vi "MecaOdometry_Reset.vi"(8 "POSE":T3={"TRANSLATION"={"X"=0.0, "Y"=0.0}, "ROTATION"={"VALUE"=0.0, "COS"=1.0, "SIN"=0.0}} {"ROTATION"."SIN" format="%13.4f"; "ROTATION"."COS" format="%13.4f"; "ROTATION"."VALUE" format="%13.4f"; "TRANSLATION"."Y" format="%14.3f"; "TRANSLATION"."X" format="%14.3f"}, 9 "WheelPositions":T1 {"RearRight" format="%19.3f"; "RearLeft" format="%19.3f"; "FrontRight" format="%19.3f"; "FrontLeft" format="%19.3f"}, 10 "GyroOffset":T5 {"SIN" format="%13.4f"; "COS" format="%13.4f"; "VALUE" format="%13.4f"}, 11 "in MECA_DRIVE_ODOMETRY":T2={"POSE"={"TRANSLATION"={"X"=0.0, "Y"=0.0}, "ROTATION"={"VALUE"=0.0, "COS"=1.0, "SIN"=0.0}}, "GyroOffset"={"VALUE"=0.0, "COS"=0.0, "SIN"=0.0}, "PreviousAngle"={"VALUE"=0.0, "COS"=0.0, "SIN"=0.0}, "Kinematics"={"FrontLeft"={"X"=0.0, "Y"=0.0}, "FrontRight"={"X"=0.0, "Y"=0.0}, "RearLeft"={"X"=0.0, "Y"=0.0}, "RearRight"={"X"=0.0, "Y"=0.0}, "InverseKinematics"=[[0.0, 1.0, -1.0, 0.0], [0.0, 1.0, 1.0, 0.0], [0.0, 1.0, 1.0, 0.0], [0.0, 1.0, -1.0, 0.0]], "ForwardKinematics"=[[0.0, 1.0, -1.0, 0.0], [0.0, 1.0, 1.0, 0.0], [0.0, 1.0, 1.0, 0.0], [0.0, 1.0, -1.0, 0.0]], "PrevCoR"={"X"=0.0, "Y"=0.0}}, "PreviousWheelPositions"={"FrontLeft"=0.0, "FrontRight"=0.0, "RearLeft"=0.0, "RearRight"=0.0, "P"=FALSE}} {"PreviousWheelPositions"."RearRight" format="%19.3f"; "PreviousWheelPositions"."RearLeft" format="%19.3f"; "PreviousWheelPositions"."FrontRight" format="%19.3f"; "PreviousWheelPositions"."FrontLeft" format="%19.3f"; "Kinematics"."PrevCoR"."Y" format="%14.3f"; "Kinematics"."PrevCoR"."X" format="%14.3f"; "Kinematics"."RearRight"."Y" format="%14.3f"; "Kinematics"."RearRight"."X" format="%14.3f"; "Kinematics"."RearLeft"."Y" format="%14.3f"; "Kinematics"."RearLeft"."X" format="%14.3f"; "Kinematics"."FrontRight"."Y" format="%14.3f"; "Kinematics"."FrontRight"."X" format="%14.3f"; "Kinematics"."FrontLeft"."Y" format="%14.3f"; "Kinematics"."FrontLeft"."X" format="%14.3f"; "PreviousAngle"."SIN" format="%13.4f"; "PreviousAngle"."COS" format="%13.4f"; "PreviousAngle"."VALUE" format="%13.4f"; "GyroOffset"."SIN" format="%13.4f"; "GyroOffset"."COS" format="%13.4f"; "GyroOffset"."VALUE" format="%13.4f"; "POSE"."ROTATION"."SIN" format="%13.4f"; "POSE"."ROTATION"."COS" format="%13.4f"; "POSE"."ROTATION"."VALUE" format="%13.4f"; "POSE"."TRANSLATION"."Y" format="%14.3f"; "POSE"."TRANSLATION"."X" format="%14.3f"}) -> (3 "out MECA_DRIVE_ODOMETRY":T2={"POSE"={"TRANSLATION"={"X"=0.0, "Y"=0.0}, "ROTATION"={"VALUE"=0.0, "COS"=1.0, "SIN"=0.0}}, "GyroOffset"={"VALUE"=0.0, "COS"=0.0, "SIN"=0.0}, "PreviousAngle"={"VALUE"=0.0, "COS"=0.0, "SIN"=0.0}, "Kinematics"={"FrontLeft"={"X"=0.0, "Y"=0.0}, "FrontRight"={"X"=0.0, "Y"=0.0}, "RearLeft"={"X"=0.0, "Y"=0.0}, "RearRight"={"X"=0.0, "Y"=0.0}, "InverseKinematics"=[[0.0, 1.0, -1.0, 0.0], [0.0, 1.0, 1.0, 0.0], [0.0, 1.0, 1.0, 0.0], [0.0, 1.0, -1.0, 0.0]], "ForwardKinematics"=[[0.0, 1.0, -1.0, 0.0], [0.0, 1.0, 1.0, 0.0], [0.0, 1.0, 1.0, 0.0], [0.0, 1.0, -1.0, 0.0]], "PrevCoR"={"X"=0.0, "Y"=0.0}}, "PreviousWheelPositions"={"FrontLeft"=0.0, "FrontRight"=0.0, "RearLeft"=0.0, "RearRight"=0.0, "P"=FALSE}} {"PreviousWheelPositions"."RearRight" format="%19.3f"; "PreviousWheelPositions"."RearLeft" format="%19.3f"; "PreviousWheelPositions"."FrontRight" format="%19.3f"; "PreviousWheelPositions"."FrontLeft" format="%19.3f"; "Kinematics"."PrevCoR"."Y" format="%14.3f"; "Kinematics"."PrevCoR"."X" format="%14.3f"; "Kinematics"."RearRight"."Y" format="%14.3f"; "Kinematics"."RearRight"."X" format="%14.3f"; "Kinematics"."RearLeft"."Y" format="%14.3f"; "Kinematics"."RearLeft"."X" format="%14.3f"; "Kinematics"."FrontRight"."Y" format="%14.3f"; "Kinematics"."FrontRight"."X" format="%14.3f"; "Kinematics"."FrontLeft"."Y" format="%14.3f"; "Kinematics"."FrontLeft"."X" format="%14.3f"; "PreviousAngle"."SIN" format="%13.4f"; "PreviousAngle"."COS" format="%13.4f"; "PreviousAngle"."VALUE" format="%13.4f"; "GyroOffset"."SIN" format="%13.4f"; "GyroOffset"."COS" format="%13.4f"; "GyroOffset"."VALUE" format="%13.4f"; "POSE"."ROTATION"."SIN" format="%13.4f"; "POSE"."ROTATION"."COS" format="%13.4f"; "POSE"."ROTATION"."VALUE" format="%13.4f"; "POSE"."TRANSLATION"."Y" format="%14.3f"; "POSE"."TRANSLATION"."X" format="%14.3f"})   [LabVIEW 2019, in "Trajectory_Library.lvlib"]
doc: "Resets the robot's position on the field.\n\nThe gyroscope angle does not need to be reset here on the user's robot code. The library automatically takes care of offsetting the gyro angle.\n \nParameters\n - MecaDriveOdometry - Data structure\n - gyroOffset - The angle reported by the gyroscope.\n - wheelPositions -- The distances driven by each wheel.\n - pose - The position on the field that your robot is at. (Meters)\n \nReturns:\n - MecaDriveOdometry - Updated ata structure"
uses:
  Trajectory_Library.lvlib
  TypeDef/TRANSLATION2D.ctl
  TypeDef/ROTATION2D.ctl
  TypeDef/POSE2D.ctl
  TypeDef/MECA_DRIVE_ODOMETRY.ctl
  <vilib>/Analysis/Matrix/Datatypes/RealMatrix.ctl
  <vilib>/Analysis/Matrix/NI_Matrix.lvlib
  TypeDef/MECA_DRIVE_KINEMATICS.ctl
  TypeDef/MECA_WHEEL_POSITIONS.ctl
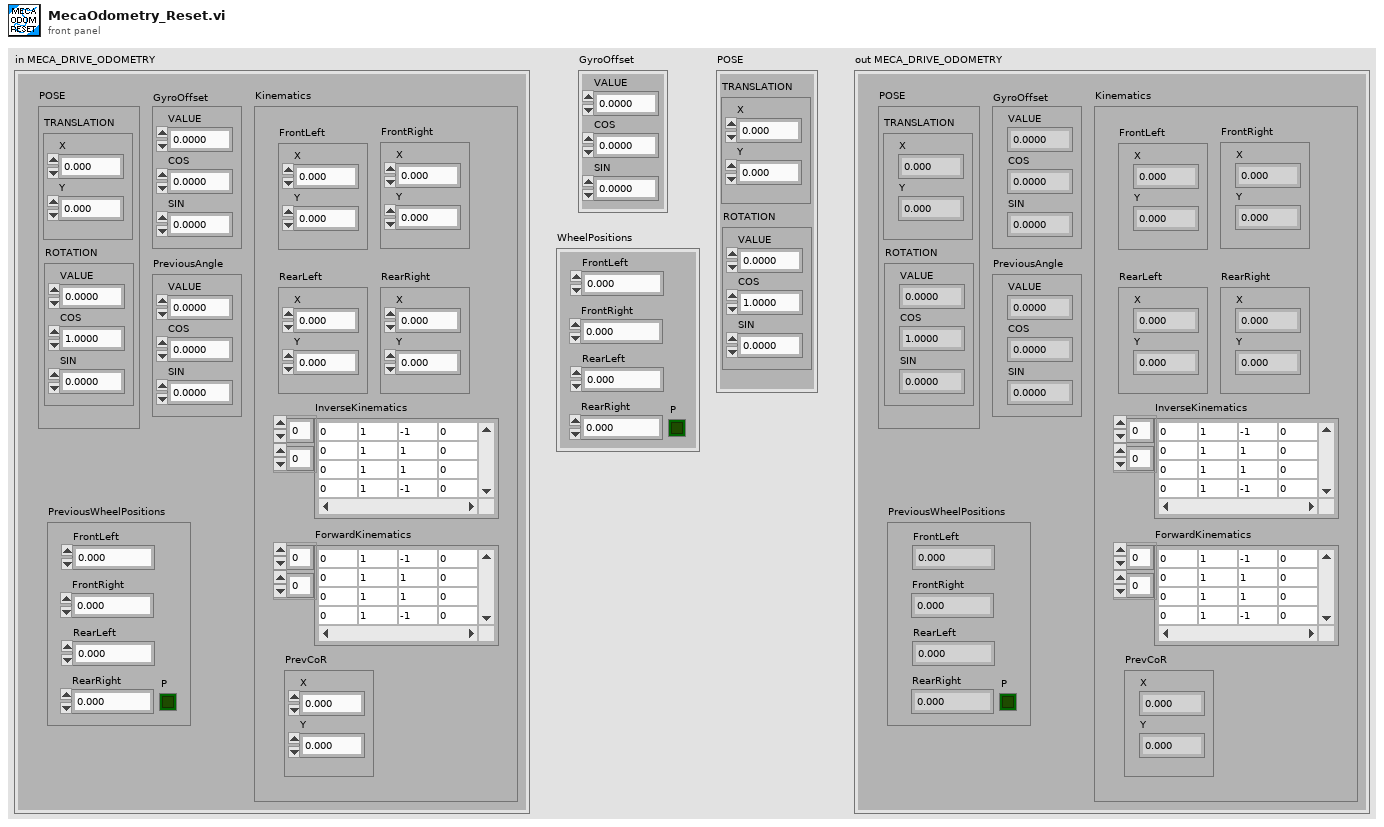
[diagram p1: front panel]
types:
  T1 = typedef "Trajectory_Library.lvlib/MECA_WHEEL_POSITIONS.ctl" = cluster{"FrontLeft":dbl, "FrontRight":dbl, "RearLeft":dbl, "RearRight":dbl, "P":bool}
  T2 = typedef "Trajectory_Library.lvlib/MECA_DRIVE_ODOMETRY.ctl" = cluster{"POSE":T3, "GyroOffset":T5, "PreviousAngle":T5, "Kinematics":T6, "PreviousWheelPositions":T1}
  T3 = typedef "Trajectory_Library.lvlib/POSE2D.ctl" = cluster{"TRANSLATION":T4, "ROTATION":T5}
  T4 = typedef "Trajectory_Library.lvlib/TRANSLATION2D.ctl" = cluster{"X":dbl, "Y":dbl}
  T5 = typedef "Trajectory_Library.lvlib/ROTATION2D.ctl" = cluster{"VALUE":dbl, "COS":dbl, "SIN":dbl}
  T6 = typedef "Trajectory_Library.lvlib/MECA_DRIVE_KINEMATICS.ctl" = cluster{"FrontLeft":T4, "FrontRight":T4, "RearLeft":T4, "RearRight":T4, "InverseKinematics":T7, "ForwardKinematics":T7, "PrevCoR":T4}
  T7 = typedef "NI_Matrix.lvlib/RealMatrix.ctl" = dbl[][]
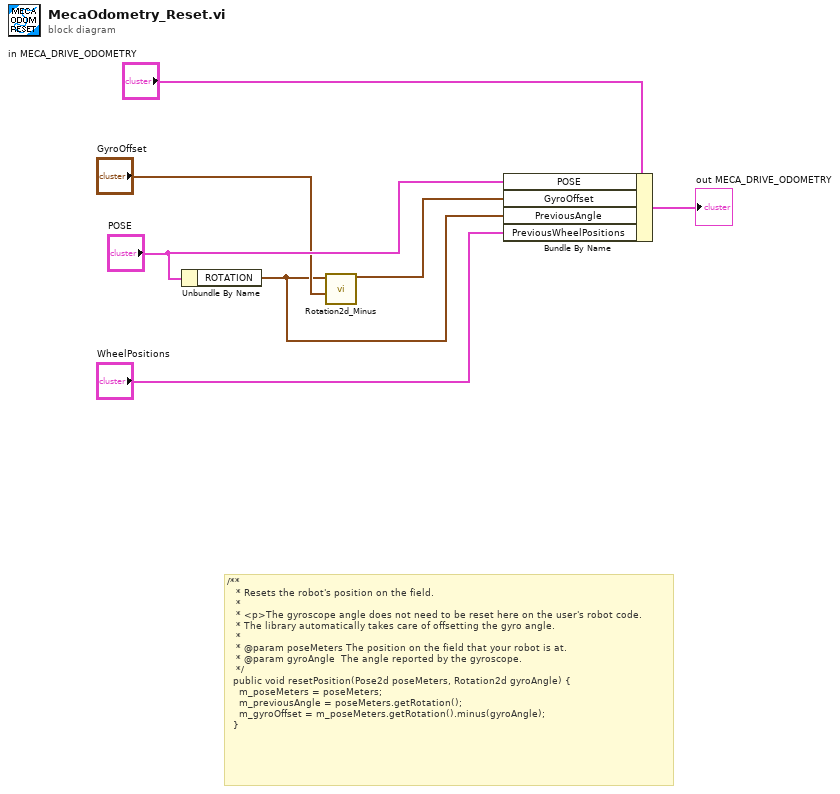
[diagram p0: block diagram]
diagram:
  # "/**\n   * Resets the robot's position on the field.\n   *\n   * <p>The gyroscope angle does not need to be reset here on the user's robot code.\n   * The library automatically takes care of offsetting the gyro angle.\n   *\n   * @param poseMeters The position on the field that your robot is at.\n   * @param gyroAngle  The angle reported by the gyroscope.\n   */\n  public void resetPosition(Pose2d poseMeters, Rotation2d gyroAngle) {\n    m_poseMeters = poseMeters;\n    m_previousAngle = poseMeters.getRotation();\n    m_gyroOffset = m_poseMeters.getRotation().minus(gyroAngle);\n  }"
  n1 = Unbundle By Name("POSE") -> ("ROTATION"=w3:T5)
  n2 = call "Rotation2d_Minus.vi"("other ROTATION"="GyroOffset", "in ROTATION"=w3) -> ("out ROTATION"=w4:T5)  [unwired: 9 in]
  n3 = Bundle By Name(cluster="in MECA_DRIVE_ODOMETRY", "POSE"="POSE", "GyroOffset"=w4, "PreviousAngle"=w3, "PreviousWheelPositions"="WheelPositions") -> (→"out MECA_DRIVE_ODOMETRY":T2)
